vi "Open PSP library.vi"(8 "error in (no error)":errorcluster, 11 "Refnum in":refnum<k21>) -> (0 "error out":errorcluster, 2 "Variables":refnum<k21>[](array[refnum]), 3 "CVT Array":T1[](array[typedef]))   [LabVIEW 2019]
uses:
  <vilib>/NI/Current Value Table/Type Defs/Single Tag.ctl
  <vilib>/NI/Current Value Table/Type Defs/Data Types.ctl
  <resource>/objmgr/ni.var.rc
  <vilib>/NI/Current Value Table/Current Value Table.lvlib
  <vilib>/Utility/Data Type/NI_Data Type.lvlib
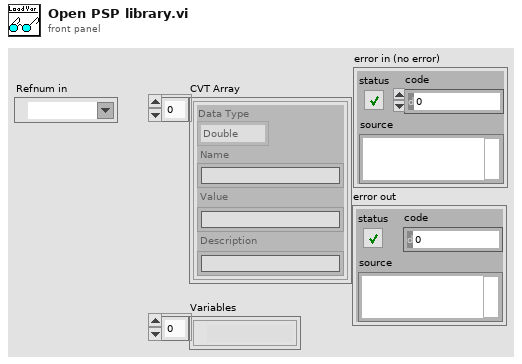
[diagram p1: front panel]
types:
  T1 = typedef "Current Value Table.lvlib/Single Tag.ctl" = cluster{"Data Type":T2, "Name":string, "Value":string, "Description":string}
  T2 = typedef "Current Value Table.lvlib/Data Types.ctl" = enum16{"Double", "Single", "I64", "I32", "I16", "I8", "U64", "U32", "U16", "U8", "String", "Boolean", "Array of U8", "Array of U16", "Array of U32", "Array of U64", "Array of I64", "Array of I32", "Array of I16", "Array of I8", "Array of Double", "Array of Single", "Array of Boolean", "Array of String"}
  T3 = cluster{"Read Access":enum8{"Allowed", "Required", "None"}, "Write Access":enum8{"Allowed", "Required", "None"}}
  T4 = typedef "NI_Data Type.lvlib/Data Type.ctl" = enum8{"Invalid Type", "Void", "I8", "I16", "I32", "I64", "U8", "U16", "U32", "U64", "Single Float", "Double Float", "Extended Float", "Single Complex", "Double Complex", "Extended Complex", "Enum U8", "Enum U16", "Enum U32", "Enum U64", "Single Float With Unit", "Double Float With Unit", "Extended Float With Unit", "Single Complex with Unit", "Double Complex with Unit", "Extended Complex with Unit", "Boolean", "String", "Path", "Picture", "Tag", "Array", "Cluster", "Variant", "LV Variant", "Waveform", "Timestamp", "Digital Waveform", "Digital Data", "ExpressData", "Refnum", "External Data", "VI", "Poly VI", "LabVIEW Class Instance", "Fixed Point", "Set Collection", "Map Collection"}
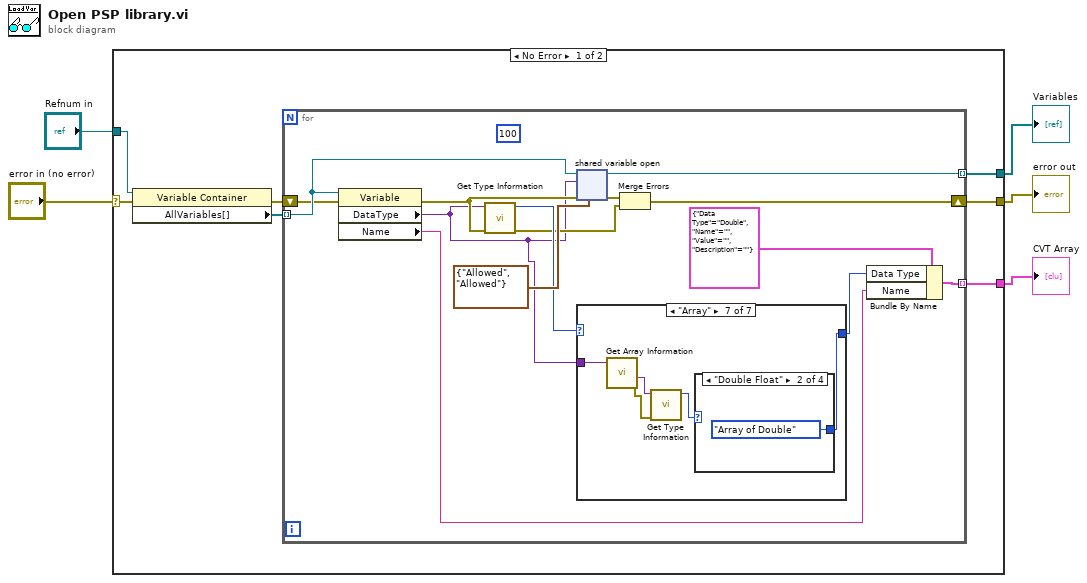
[diagram p0: block diagram]
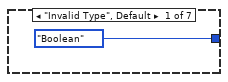
[diagram p2: hidden frame]
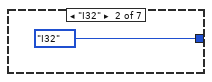
[diagram p3: hidden frame]
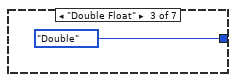
[diagram p4: hidden frame]
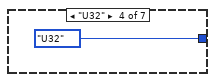
[diagram p5: hidden frame]
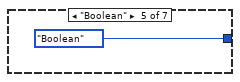
[diagram p6: hidden frame]
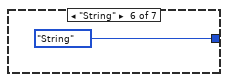
[diagram p7: hidden frame]
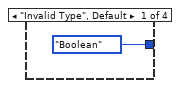
[diagram p8: hidden frame]
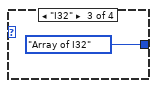
[diagram p9: hidden frame]
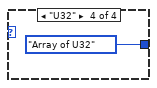
[diagram p10: hidden frame]
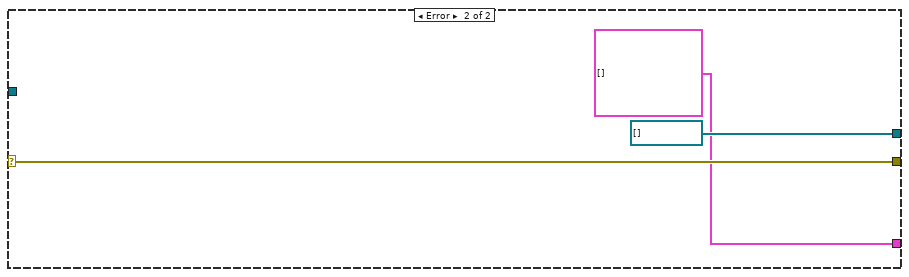
[diagram p11: hidden frame]
diagram:
  n1 = case shown="No Error" "error in (no error)" {
    selector: "error in (no error)" -> [w6 w43]
    tunnel: [w12 T1[] []] -> w5
    tunnel: [w11 refnum<k21>[] []] -> w4
    tunnel: "Refnum in" -> [w9 _]
    tunnel: [w7 w43] -> w2
    frame No Error {
      n2 = property class="Variable Container"(reference=w9, error in=w6) -> (error out=w8:errorcluster, "AllVariables[]"=w10:refnum<k21>[])  [unwired: 1 out]
      n3 = for {
        tunnel: w10 -> [w25] mode=indexing
        tunnel: [w14] -> w11 mode=indexing
        tunnel: [w20] -> w12 mode=indexing
        shift-right: [w15] -> w7
        shift-left: w8 -> [w16]
        (unwired) 100 ("timeout ms")
        n4 = property class="Variable"(reference=w25, error in=w16) -> (error out=w19:errorcluster, "DataType"=w13:variant, "Name"=w23:string)  [unwired: 1 out]
        n5 = call <vilib>:"Get Type Information.vi"("error in (no error)"=w19, "variant"=w13) -> ("error out"=w17:errorcluster, "type"=w22:T4)  [unwired: 5 in, 3 out]
        n6 = shared-variable-open(w25, w19, w13, T3 {"Read Access"=enum."Allowed", "Write Access"=enum."Allowed"} ("access")) -> (w14:refnum<k21>, w18:errorcluster)  [unwired: 1 in]
        n7 = case shown="\"Array\"" w22 {
          tunnel: [Data_Types."Boolean" ("Data Type") Data_Types."I32" ("Data Type") Data_Types."Double" ("Data Type") Data_Types."U32" ("Data Type") Data_Types."Boolean" ("Data Type") Data_Types."String" ("Data Type") w33] -> w21
          tunnel: w13 -> [_ _ _ _ _ _ w37]
          frame "Invalid Type", Default {
          }
          frame "I32" {
          }
          frame "Double Float" {
          }
          frame "U32" {
          }
          frame "Boolean" {
          }
          frame "String" {
          }
          frame "Array" {
            n8 = call <vilib>:"Get Array Information.vi"("variant"=w37) -> ("error out"=w35:errorcluster, "array element data type"=w36:variant)  [unwired: 7 in, 2 out]
            n9 = call <vilib>:"Get Type Information.vi"("error in (no error)"=w35, "variant"=w36) -> ("type"=w34:T4)  [unwired: 5 in, 4 out]
            n10 = case shown="\"Double Float\"" w34 {
              tunnel: [Data_Types."Boolean" ("Data Type") Data_Types."Array of Double" ("Data Type") Data_Types."Array of I32" ("Data Type") Data_Types."Array of U32" ("Data Type")] -> w33
              frame "Invalid Type", Default {
              }
              frame "Double Float" {
              }
              frame "I32" {
              }
              frame "U32" {
              }
            }
          }
        }
        n11 = Merge Errors(w18, w17) -> (w15:errorcluster)
        n12 = Bundle By Name(cluster=T1 {"Data Type"=enum."Double", "Name"="", "Value"="", "Description"=""} ("Tag"), "Data Type"=w21, "Name"=w23) -> (w20:T1)
      }
    }
    frame Error {
    }
  }
  "CVT Array" <- w5
  "Variables" <- w4
  "error out" <- w2
